vi "unary_client.vi"() -> ()   [LabVIEW 2019]
uses:
  Generated_client/RPC Messages/routeguide_Color.ctl
  Generated_client/RPC Messages/routeguide_request.ctl
  Generated_client/Generated_client.lvlib
panel:
  out "response_color":T1
  out "response_message":string
  out "response_number":i32
  in  "request_color":T1=enum."GREEN"
  in  "request_message":string="Hi"
  in  "request_number":i32=101
  out "error out":errorcluster
  in  "error in":errorcluster
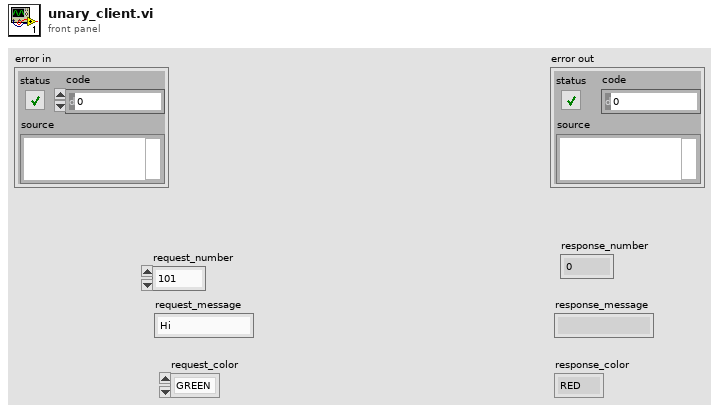
[diagram p1: front panel]
types:
  T1 = typedef "Generated_client.lvlib/routeguide_Color.ctl" = enum32{"RED", "GREEN", "BLUE"}
  T2 = typedef "Generated_client.lvlib/routeguide_request.ctl" = cluster{"request_number":i32, "request_message":string, "request_color":T1}
  T3 = typedef "grpc-lvsupport-release.lvlib/grpcId.ctl" = u64
  T4 = typedef "Generated_client.lvlib/routeguide_response.ctl" = cluster{"response_number":i32, "response_message":string, "response_color":T1}
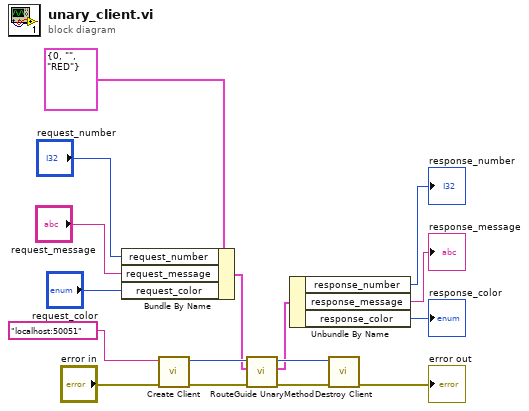
[diagram p0: block diagram]
diagram:
  n1 = Bundle By Name(cluster=T2 {"request_number"=0, "request_message"="", "request_color"=enum."RED"} ("routeguide_request"), "request_number"="request_number", "request_message"="request_message", "request_color"="request_color") -> (w5:T2)
  n2 = call "Create Client.vi"("error in"="error in", "address"="localhost:50051") -> ("error out"=w14:errorcluster, "gRPC ID Out"=w16:T3)  [unwired: 8 in]
  n3 = call "RouteGuide UnaryMethod.vi"("error in"=w14, "Request Data"=w5, "gRPC ID"=w16) -> ("error out"=w13:errorcluster, "Response Data"=w4:T4, "gRPC ID out"=w15:T3)  [unwired: 6 in]
  n4 = Unbundle By Name(w4) -> ("response_number"=→"response_number":i32, "response_message"=→"response_message":string, "response_color"=→"response_color":T1)
  n5 = call "Destroy Client.vi"("error in"=w13, "gRPC ID"=w15) -> ("error out"=→"error out":errorcluster)  [unwired: 9 in]
